vi "inclineAquire.vi"(8 "error in (no error)":errorcluster, 10 "Negative Incline":dbl, 11 "VISA Refnum in":refnum<visa-resource-name>) -> (0 "error out":errorcluster, 3 "Incline Out":dbl)   [LabVIEW 2018]
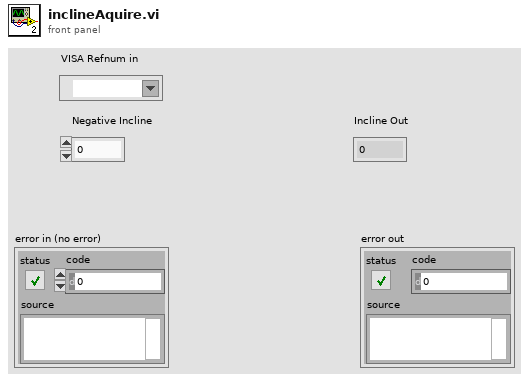
[diagram p1: front panel]
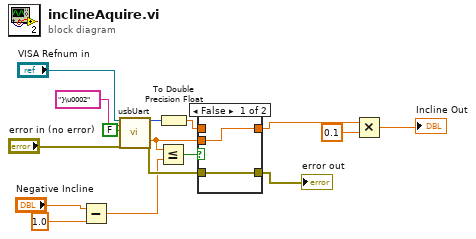
[diagram p0: block diagram]
diagram:
  n1 = Subtract(x="Negative Incline", y=1.0) -> (x-y=w3:dbl)
  n2 = call "usbUart.vi"("VISA resource name"="VISA Refnum in", "write buffer"="}\u0002" ("write buffer 2"), "sdFeature"=FALSE, "error in (no error)"="error in (no error)") -> ("number[0]"=w14:u32, "negative incline"=w15:dbl, "error out"=w9:errorcluster)  [unwired: 13 out]
  n3 = Less Or Equal?(x=w15, y=w3) -> (x <= y?=w12:bool)
  n4 = To Double Precision Float(number=w14) -> (double precision float=w13:dbl)
  n5 = case shown="False" w12 {
    tunnel: w15 -> [w18 _]
    tunnel: w13 -> [_ w20]
    tunnel: [w18 w20] -> w6
    tunnel: w9 -> [w17 w19]
    tunnel: [w17 w19] -> w8
    frame False {
    }
    frame True {
    }
  }
  "error out" <- w8
  n6 = Multiply(x=w6, y=0.1) -> (x*y=→"Incline Out":dbl)
